vi "AutoDetector_RunResult.vi"(8 "Error In":errorcluster, 9 "Correct Run Bias Reached":bool, 10 "Optimized DV Value":u32, 11 "Auto-DV Info In":T2) -> (0 "Error Out":errorcluster, 2 "Next State":T1=enum."Get Cal Files", 3 "Auto-DV Info Out":T2)   [LabVIEW 2015]
uses:
  Controls/Auto-Detector Bias Info.ctl
  Controls/Auto-Detector Peak Info.ctl
  Type/_CalibrationStep.ctl
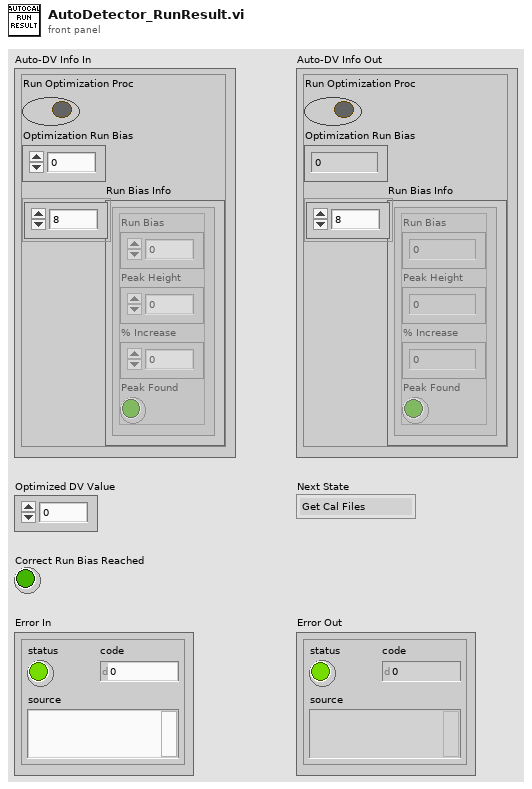
[diagram p1: front panel]
types:
  T1 = typedef "_CalibrationStep.ctl" = enum16{"Export Optimization", "Get Cal Files", "Read Q1 Method", "Acquire Q1 Data", "Process Q1 Data", "Generate Report", "Prepare For Q2 Cal", "Read Q2 Method", "Acquire Q2 Data", "Process Q2 Data", "Done", "Pause"}
  T2 = typedef "Auto-Detector Bias Info.ctl" = cluster{"Run Optimization Proc":bool, "Optimization Run Bias":u32, "Run Bias Info":T3[]}
  T3 = typedef "Auto-Detector Peak Info.ctl" = cluster{"Run Bias":u32, "Peak Height":dbl, "% Increase":dbl, "Peak Found":bool}
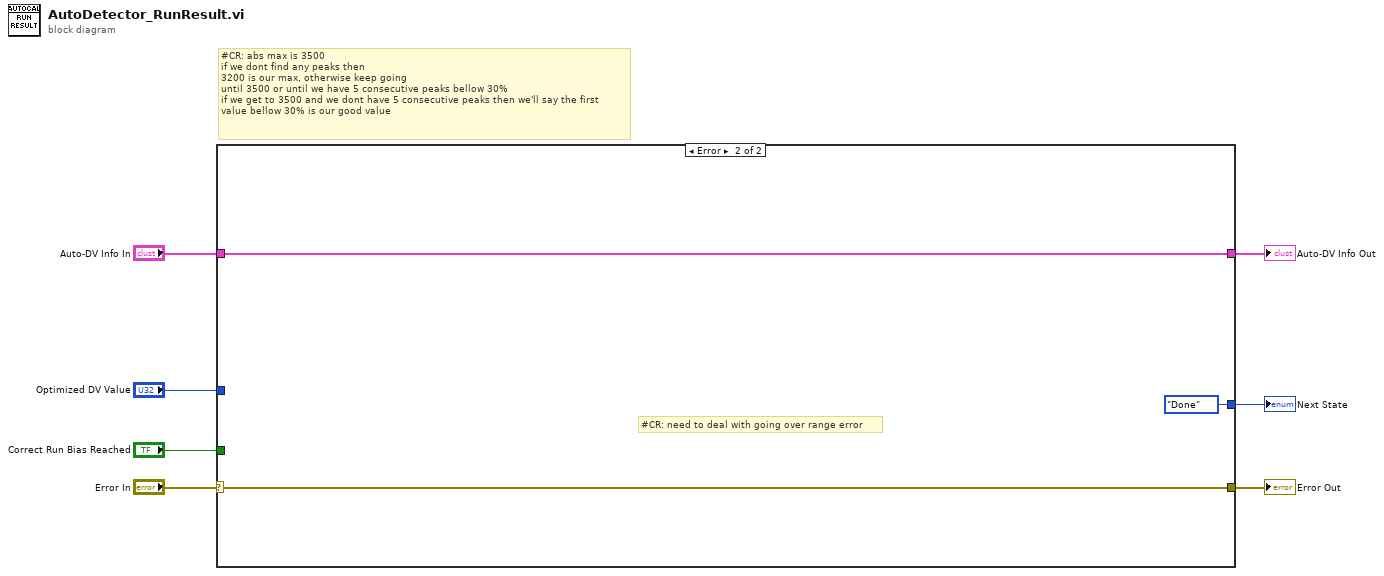
[diagram p0: block diagram]
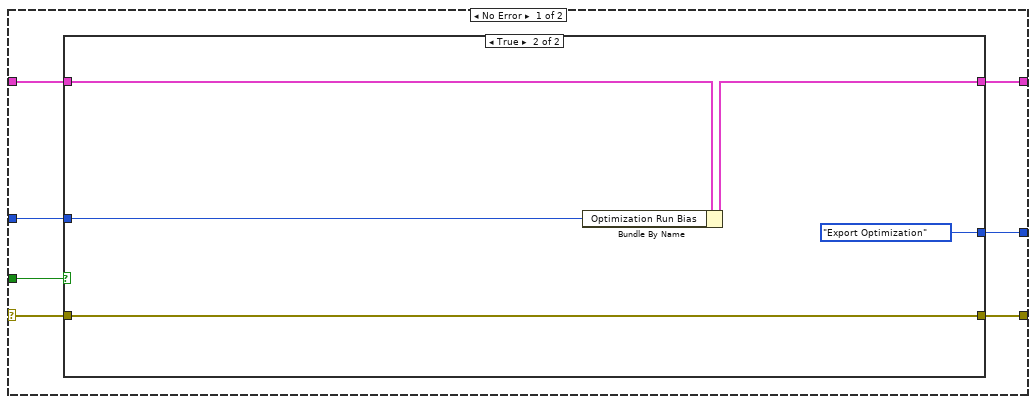
[diagram p2: hidden frame]
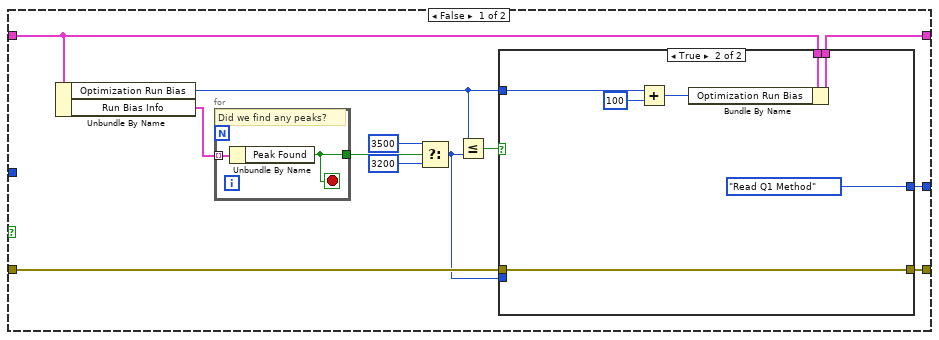
[diagram p3: hidden frame]
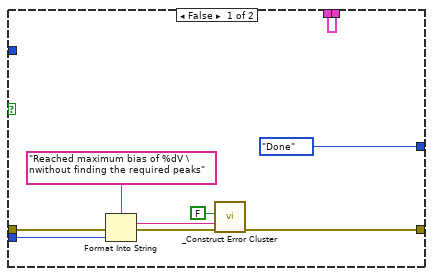
[diagram p4: hidden frame]
diagram:
  # "#CR: abs max is 3500\nif we dont find any peaks then\n3200 is our max, otherwise keep going\nuntil 3500 or until we have 5 consecutive peaks bellow 30%\nif we get to 3500 and we dont have 5 consecutive peaks then we'll say the first\nvalue bellow 30% is our good value"
  n1 = case shown="Error" "Error In" {
    selector: "Error In" -> [w9 w52]
    tunnel: [w8 w52] -> w6
    tunnel: [w11 w51] -> w5
    tunnel: "Auto-DV Info In" -> [w12 w51]
    tunnel: "Optimized DV Value" -> [w13 _]
    tunnel: "Correct Run Bias Reached" -> [w14 _]
    tunnel: [w10 _CalibrationStep."Done" ("Next State")] -> w1
    frame No Error {
      n2 = case shown="True" w14 {
        tunnel: w13 -> [_ w46]
        tunnel: w12 -> [w26 w49]
        tunnel: [w25 w47] -> w11
        tunnel: [w22 _CalibrationStep."Export Optimization" ("Next State")] -> w10
        tunnel: w9 -> [w21 w45]
        tunnel: [w20 w45] -> w8
        frame False {
          n3 = Unbundle By Name(w26) -> ("Optimization Run Bias"=w23:u32, "Run Bias Info"=w19:T3[])
          n4 = for {
            tunnel: w19 -> [w28] mode=indexing
            tunnel: [w27] -> w16
            stop <- w27 stop-if-true
            # "Did we find any peaks?"
            n5 = Unbundle By Name(w28) -> ("Peak Found"=w27:bool)
          }
          n6 = Select(t=u32 3500 ("y"), s=w16, f=u32 3200 ("y")) -> (s? t:f=w15:u32)
          n7 = Less Or Equal?(x=w23, y=w15) -> (x <= y?=w24:bool)
          n8 = case shown="True" w24 {
            tunnel: w26 -> [w37 w44]
            tunnel: [w37 w43] -> w25
            tunnel: w23 -> [_ w42]
            tunnel: [_CalibrationStep."Done" ("t") _CalibrationStep."Read Q1 Method" ("Next State")] -> w22
            tunnel: w21 -> [w30 w38]
            tunnel: [w34 w38] -> w20
            tunnel: w15 -> [w33 _]
            frame False {
              n9 = Format Into String(format string="Reached maximum bias of %dV \nwithout finding the required peaks", error in=w30, w33) -> (resulting string=w31:string, error out=w29:errorcluster)  [unwired: 1 in]
              n10 = call "_Construct Error Cluster.vi"("error in"=w29, "reason"=w31, "CallingChain? (T)"=FALSE) -> ("error out"=w34:errorcluster)  [unwired: 4 in]
            }
            frame True {
              n11 = Add(x=w42, y=u32 100) -> (x+y=w41:u32)
              n12 = Bundle By Name(cluster=w44, "Optimization Run Bias"=w41) -> (w43:T2)
            }
          }
        }
        frame True {
          n13 = Bundle By Name(cluster=w49, "Optimization Run Bias"=w46) -> (w47:T2)
        }
      }
    }
    frame Error {
      # "#CR: need to deal with going over range error"
    }
  }
  "Error Out" <- w6
  "Auto-DV Info Out" <- w5
  "Next State" <- w1
